vi "Subtask1_Move.vi"   [LabVIEW 2016]
uses:
  <vilib>/NXT/Subs/LVHSConnector.ctl
  <vilib>/NXT/LegoClasses/BrickReference/BrickReference.lvclass
  <vilib>/NXT/Block Support/NXT_OutputPort.ctl
  <vilib>/NXT/NXTIO Xnodes/NXTIONodeSubVIs/NXTMoveMotors.vi
  <vilib>/NXT/Dual Mode Library/Waits/Wait_Num.vi
  <vilib>/NXT/NXTIO Xnodes/AddressXNode/NXTIOAddress.xnode
  <vilib>/NXT/NXTIO Xnodes/NXTIOXNode/NXTIO.xnode
types:
  T1 = typedef "LVHSConnector.ctl" = refnum<class "BrickReference.lvclass">
  T2 = typedef "NXT_OutputPort.ctl" = u8
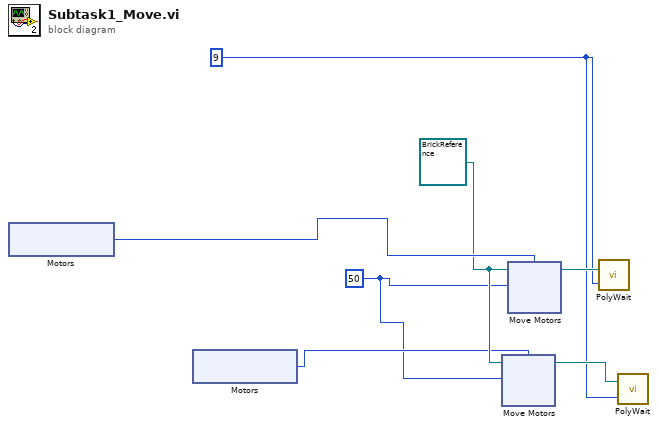
[diagram p0: block diagram]
diagram:
  w1 = 9
  w5 = T1 refnum ("NXT/EV3")
  w2 = i8 50 ("Speed 1")
  n1 = xnode "Motors"() -> ("Motor"=w7:T2)
  n2 = xnode "Motors"() -> ("Motor"=w4:T2)
  n3 = xnode "Move Motors"("Power/Speed 1"=w2, "Motors"=w4, "NXT/EV3"=w5) -> ("NXT/EV3"=w3:T1)
  n4 = xnode "Move Motors"("Power/Speed 1"=w2, "Motors"=w7, "NXT/EV3"=w5) -> ("NXT/EV3"=w6:T1)
  n5 = call-poly <vilib>:"PolyWait.vi"("Time (1 sec)"=w1, "NXT/EV3"=w6) -> ()  [unwired: 2 in, 1 out]
  n6 = call-poly <vilib>:"PolyWait.vi"("Time (1 sec)"=w1, "NXT/EV3"=w3) -> ()  [unwired: 2 in, 1 out]
